vi "NanotecSMCPD.check axis reference move.vi"(0 "i ref in":refnum<vi>, 1 "axis":i32, 3 "ms timeout (10000)":i32=10000, 5 "error in (no error)":errorcluster) -> (14 "i ref out":refnum<vi>, 17 "timed out":bool, 19 "error out":errorcluster)   [LabVIEW 2014, in "NanotecSMCPD.lvlib"]
doc: "Checks, if a reference move is finished. This method does not query the instrument, but decides on the basis of \n\n1) the \"in position\" bit of the status word of the MotorBase class.\n2) the \"referencing\" attribute of THIS class.\n\nFor proper operation, the \"get axis status\" method of THIS class must be executed prior to executing this method."
uses:
  NanotecSMCPD.lvlib
  CSCore/CSSystem/CoreDefs/CoreDefs.error_type.ctl
  CSCore/CSSystem/CoreDefs/CoreDefs.error_severity.ctl
  CSCore/CSApplicationBaseClasses/MotorBase/MotorBase.statusType.ctl
  CSCore/CSApplicationBaseClasses/MotorBase/MotorBase.directionType.ctl
  CSCore/CSApplicationBaseClasses/MotorBase/MotorBase.serviceType.ctl
  CSlibraries/UtilityLib/UtilityLib.valueStatus.ctl
  CSCore/CSApplicationBaseClasses/DeviceBase/DeviceBase.lvlib
  CSCore/CSApplicationBaseClasses/MotorBase/MotorBase.lvlib
  CSlibraries/UtilityLib/UtilityLib.lvlib
  CSCore/CSSystem/CoreLib/CoreLib.lvlib
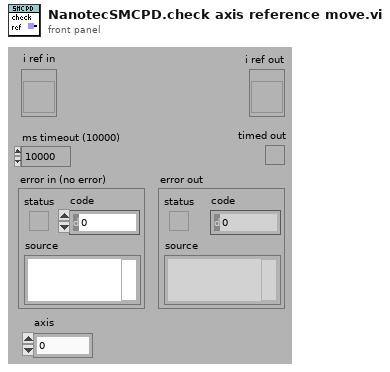
[diagram p1: front panel]
types:
  T1 = typedef "CoreDefs.error_severity.ctl" = enum16{"undefined", "information", "warning", "error", "fatal"}
  T2 = typedef "CoreDefs.error_type.ctl" = enum16{"no error", "can't load process", "can't unload process", "process does not exist", "can't install process", "can't remove process", "unknown function", "time out", "can't execute function", "duplicate queue name", "super not found", "caller queue invalid", "can't ping process", "unknown error", "VISA Error", "VISA timeout", "GPIB timeout", "GPIB error", "communication error", "data type mismatch", "can't read data from OPC server", "can't write data to OPC server", "OET error", "function not implemented", "process already exists", "invalid Shared Variable name", "error writing Shared Variable", "error reading Shared Variable", "invalid client name", "corrupt database", "unknown class", "call not authorized", "parameter out of range", "OET timeout: can't get data to modify", "invalid queue name", "requested operation incompatible with current state", "event undefined", "event disabled", "state undefined", "caller is not a friend", "EventBuilder: bad eventID", "EventBuilder: no DAQ devices", "a thread must not stop itself", "UNUSED ELEMENT4", "DiscArchiver: eventData incomplete", "DiscArchiver: eventData does not belong to run", "DiscArchiver: can't open file", "DiscArchiver: can't write to file", "DiscArchiver: available disc space low", "can't acquire semaphore", "error reading data from database", "notifier object is not existing", "can't register process", "can't unregister process", "illegal event type", "object disabled", "object already exists", "can't change state", "Instrument not found", "no connection to remote node", "invalid reference", "N/A", "UNUSED ELEMENT 1", "element not found", "illegal TCP/IP connection detected", "object does not exist", "invalid access ID", "unknown CS system", "invalid privilige", "unsupported data type", "unsupported server type", "IO server already exists", "Shared Variable already exists"}
  T3 = typedef "UtilityLib.lvlib/UtilityLib.valueStatus.ctl" = enum16{"no info available", "stand by/off", "on", "warning", "alarm/malfunction", "not implemented", "user action required", "important information", "system default", "control default", "indicator default", "button default"}
  T4 = typedef "MotorBase.lvlib/MotorBase.serviceType.ctl" = enum16{"onOff", "startVelocity", "stopVelocity", "acceleration", "rangeMin", "rangeMax", "status", "position"}
  T5 = typedef "MotorBase.lvlib/MotorBase.directionType.ctl" = enum16{"unknown", "update actual value", "update nominal value", "update both"}
  T6 = typedef "MotorBase.lvlib/MotorBase.statusType.ctl" = u32
  T7 = typedef "NanotecSMCPD.lvlib/NanotecSMCPD.i attribute.ctl" = cluster{"referencing":bool[], "stop":bool[], "AutoHalt ID":i32, "MethodQueue":refnum<queue>, "Referenced1Time?":bool[], "LastCommand ID":i32}
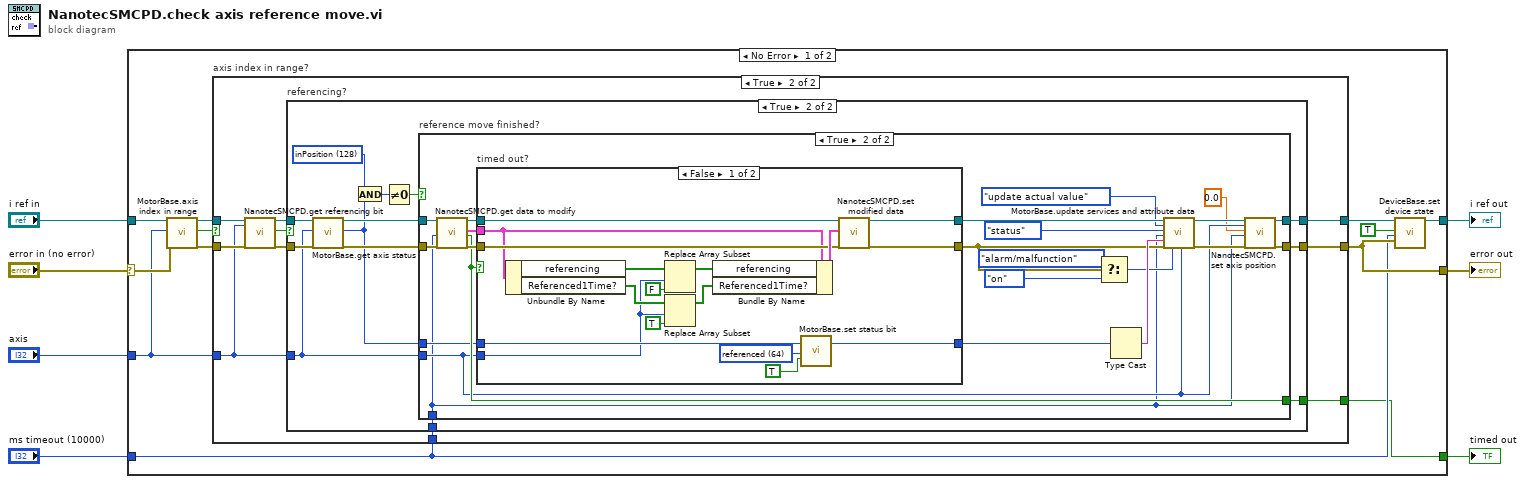
[diagram p0: block diagram]
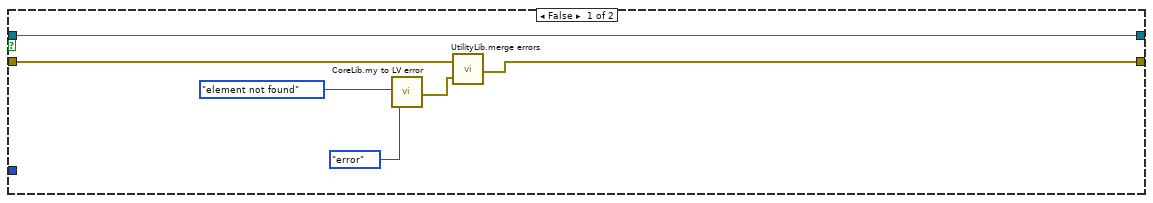
[diagram p2: hidden frame]
diagram:
  n1 = case shown="No Error" "error in (no error)" {
    selector: "error in (no error)" -> [w11 w96]
    tunnel: "ms timeout (10000)" -> [w15 _]
    tunnel: "i ref in" -> [w12 w97]
    tunnel: [w17 w96] -> w4
    tunnel: [w18 w97] -> w3
    tunnel: [w14 _] -> w2
    tunnel: "axis" -> [w8 _]
    frame No Error {
      n2 = call "MotorBase.axis index in range.vi"("i ref in"=w12, "axisIndex"=w8, "error in (no error)"=w11) -> ("i ref out"=w13:refnum<vi>, "in range"=w9:bool, "error out"=w10:errorcluster)  [unwired: 14 in]
      n3 = case "axis index in range?" shown="True" w9 {
        tunnel: w13 -> [w25 w31]
        tunnel: w10 -> [w24 w30]
        tunnel: [w23 w35] -> w17
        tunnel: [w25 w34] -> w16
        tunnel: w15 -> [_ w33]
        tunnel: [_ w32] -> w14
        tunnel: w8 -> [_ w29]
        frame False {
          n4 = call "CoreLib.my to LV error.vi"("ErrorTypes"=CoreDefs.error_type."element not found", "severityLevel"=CoreDefs.error_severity."error") -> ("myErrorCluster"=w22:errorcluster)  [unwired: 16 in, 1 out]
          n5 = call "UtilityLib.merge errors.vi"("error2 (no error)"=w22, "error1 (no error)"=w24) -> ("error out"=w23:errorcluster)
        }
        frame True {
          n6 = call "NanotecSMCPD.get referencing bit.vi"("i ref in"=w31, "axis"=w29, "error in (no error)"=w30) -> ("i ref out"=w28:refnum<vi>, "isReferencing?"=w26:bool, "error out"=w27:errorcluster)  [unwired: 14 in]
          n7 = case "referencing?" shown="True" w26 {
            tunnel: w28 -> [w37 w50]
            tunnel: w27 -> [w36 w49]
            tunnel: w29 -> [_ w40]
            tunnel: w33 -> [_ w44]
            tunnel: [w37 w43] -> w34
            tunnel: [w36 w42] -> w35
            tunnel: [_ w39] -> w32
            frame False {
            }
            frame True {
              w41 = T6 128 items=["motorEnabled"=1, "negativeLimitSwitchActive"=2, "positiveLimitSwitchActive"=4, "limitSwitchesEnabled"=8, "limitSwitchesAreNormallyClosed"=16, "moving"=32, "referenced"=64, "inPosition"=128, "reserved2"=256, "reserved3"=512, "reserved4"=1024, "reserved5"=2048, "error"=4096, "reserved6"=8192, "reserved7"=16384, "reserved8"=32768, "user defined1"=65536, "user defined2"=131072, "user defined3"=262144, "user defined4"=524288, "user defined5"=1048576, "user defined6"=2097152, "user defined7"=4194304, "user defined8"=8388608, "user defined9"=16777216, "user defined10"=33554432, "user defined11"=67108864, "user defined12"=134217728, "user defined13"=268435456, "user defined14"=536870912, "user defined15"=1073741824, "user defined16"=2147483648] ("status")
              n8 = call "MotorBase.get axis status.vi"("i ref in"=w50, "axisIndex"=w40, "error in (no error)"=w49) -> ("i ref out"=w46:refnum<vi>, "status"=w38:T6, "error out"=w45:errorcluster)  [unwired: 14 in]
              n9 = And(x=w41, y=w38) -> (x .and. y?=w48:T6)
              n10 = Not Equal To 0?(x=w48) -> (x != 0?=w47:bool)
              n11 = case "reference move finished?" shown="True" w47 {
                tunnel: w46 -> [w52 w75]
                tunnel: w45 -> [w51 w74]
                tunnel: w44 -> [_ w54]
                tunnel: [w52 w57] -> w43
                tunnel: [w51 w56] -> w42
                tunnel: w40 -> [_ w55]
                tunnel: [_ w70] -> w39
                tunnel: w38 -> [_ w69]
                frame False {
                }
                frame True {
                  n12 = call "NanotecSMCPD.get data to modify.vi"("i ref in"=w75, "ms timeout (10000)"=w54, "error in (no error)"=w74) -> ("i ref out"=w73:refnum<vi>, "i attribute"=w71:T7, "timed out"=w70:bool, "error out"=w72:errorcluster)  [unwired: 13 in]
                  n13 = case "timed out?" shown="False" w70 {
                    tunnel: [w92 w95] -> w68
                    tunnel: w73 -> [w87 w95]
                    tunnel: w72 -> [w86 w94]
                    tunnel: [w91 w94] -> w63
                    tunnel: w55 -> [w76 _]
                    tunnel: w71 -> [w81 _]
                    tunnel: w69 -> [w85 w93]
                    tunnel: [w82 w93] -> w65
                    frame False {
                      w84 = T6 64 items=["motorEnabled"=1, "negativeLimitSwitchActive"=2, "positiveLimitSwitchActive"=4, "limitSwitchesEnabled"=8, "limitSwitchesAreNormallyClosed"=16, "moving"=32, "referenced"=64, "inPosition"=128, "reserved2"=256, "reserved3"=512, "reserved4"=1024, "reserved5"=2048, "error"=4096, "reserved6"=8192, "reserved7"=16384, "reserved8"=32768, "user defined1"=65536, "user defined2"=131072, "user defined3"=262144, "user defined4"=524288, "user defined5"=1048576, "user defined6"=2097152, "user defined7"=4194304, "user defined8"=8388608, "user defined9"=16777216, "user defined10"=33554432, "user defined11"=67108864, "user defined12"=134217728, "user defined13"=268435456, "user defined14"=536870912, "user defined15"=1073741824, "user defined16"=2147483648] ("statusBit")
                      n14 = Unbundle By Name(w81) -> ("referencing"=w80:bool[], "Referenced1Time?"=w77:bool[])
                      n15 = Replace Array Subset(array=w80, new element=FALSE ("new element/subarray"), index=w76) -> (w89:bool[])
                      n16 = Replace Array Subset(array=w77, new element=TRUE ("new element/subarray"), index=w76) -> (w78:bool[])
                      n17 = Bundle By Name(cluster=w81, "referencing"=w89, "Referenced1Time?"=w78) -> (w88:T7)
                      n18 = call "MotorBase.set status bit.vi"("status"=w85, "statusBit"=w84, "setBit"=TRUE) -> ("status out"=w82:T6)  [unwired: 16 in]
                      n19 = call "NanotecSMCPD.set modified data.vi"("i ref in"=w87, "i attribute"=w88, "error in (no error)"=w86) -> ("i ref out"=w92:refnum<vi>, "error out"=w91:errorcluster)  [unwired: 15 in]
                    }
                    frame True {
                    }
                  }
                  n20 = Select(t=UtilityLib.valueStatus."alarm/malfunction" ("quality"), s=w63, f=UtilityLib.valueStatus."on" ("quality")) -> (s? t:f=w60:T3)
                  n21 = Type Cast(x=w65) -> (*(type *) &x=w64:string)  [unwired: 1 in]
                  n22 = call "MotorBase.update services and attribute data.vi"("i ref in"=w68, "direction"=MotorBase.directionType."update actual value", "service"=MotorBase.serviceType."status", "ms timeout (10000)"=w54, "value"=w64, "error in (no error)"=w63, "quality"=w60, "axisNumber"=w55) -> ("i ref out"=w59:refnum<vi>, "error out"=w58:errorcluster)  [unwired: 9 in, 1 out]
                  n23 = call "NanotecSMCPD.set axis position.vi"("i ref in"=w59, "axis"=w55, "position"=0.0, "ms timeout (10000)"=w54, "error in (no error)"=w58) -> ("i ref out"=w57:refnum<vi>, "error out"=w56:errorcluster)  [unwired: 12 in, 1 out]
                }
              }
            }
          }
        }
      }
      n24 = call "DeviceBase.set device state.vi"("i ref in"=w16, "implicit"=TRUE, "ms timeout (10000)"=w15, "device error"=w17) -> ("i ref out"=w18:refnum<vi>)  [unwired: 13 in, 2 out]
    }
    frame Error {
    }
  }
  "error out" <- w4
  "i ref out" <- w3
  "timed out" <- w2
